vi "SaveCycleSweep.vi"(5 "Area":dbl=1.0, 6 "JunctionName":string, 7 "SideLength":dbl=1.0, 8 "UiDefinition 2":T3, 9 "InfoCluster":T1, 10 "appended array":dbl[][](array[numeric])) -> (0 "error out":errorcluster)   [LabVIEW 2020]
uses:
  UIReferences.ctl
  D:/LabviewDXFViewer/LabviewDXFViewer/bin/Release/LabviewDXFViewer.exe
  LabviewDXFViewer/bin/Release/LabviewDXFViewer.exe
  Keithley_Subs/CapacitanceInfos.ctl
  Keithley_Subs/CapacitanceRecord.ctl
  <vilib>/httpClient/POSTBuffer.vi
  <vilib>/httpClient/LabVIEWHTTPClient.lvlib
panel:
  in  "Cluster 3":T4
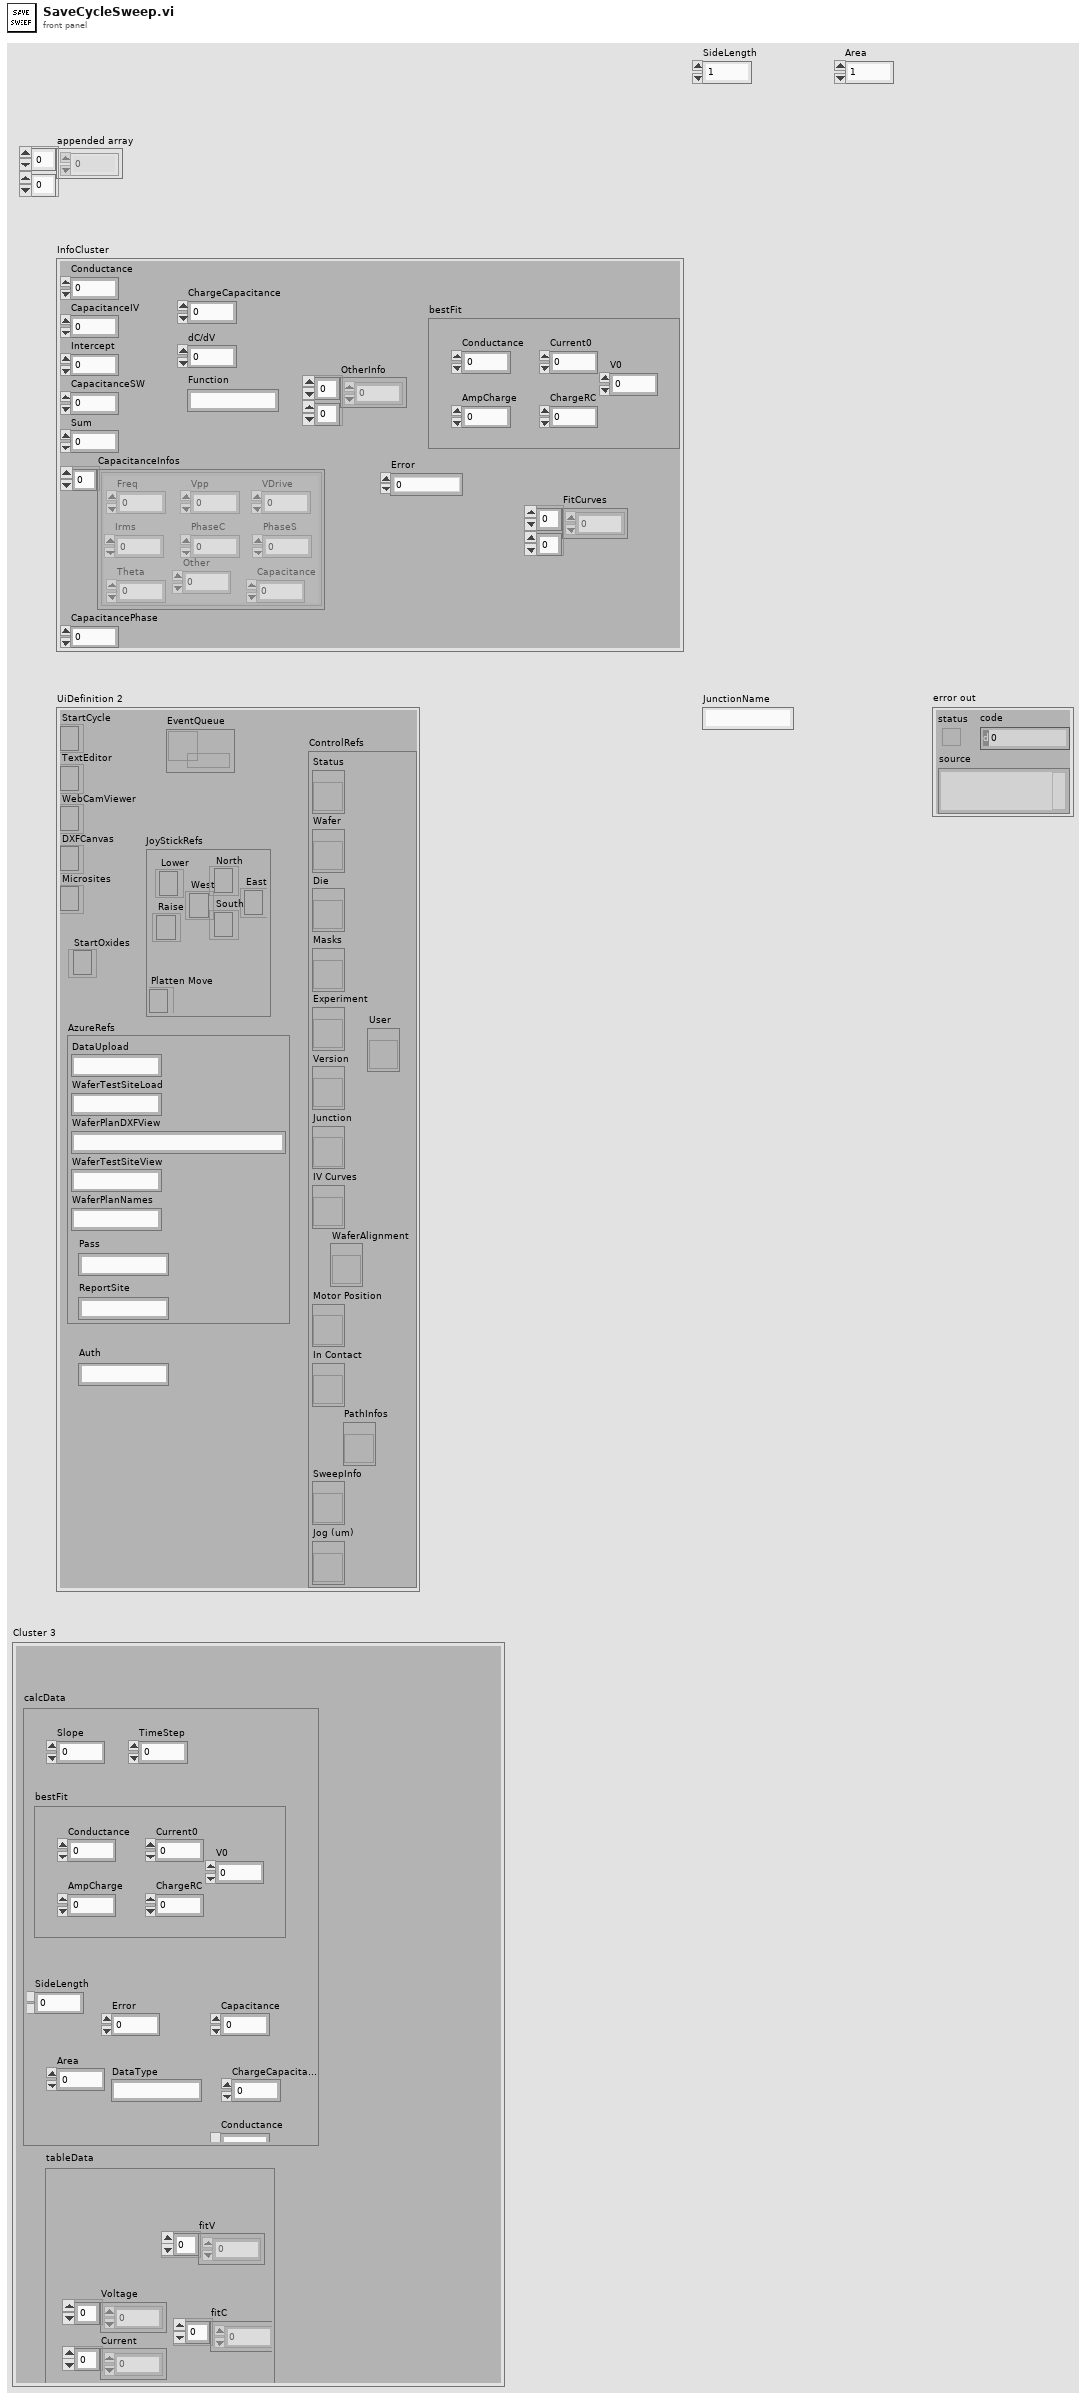
[diagram p1: front panel]
types:
  T1 = typedef "CapacitanceInfos.ctl" = cluster{"Conductance":dbl, "CapacitanceIV":dbl, "Intercept":dbl, "CapacitanceSW":dbl, "Sum":dbl, "CapacitanceInfos":T2[], "CapacitancePhase":dbl, "dC/dV":dbl, "Function":string, "OtherInfo":dbl[][], "ChargeCapacitance":dbl, "FitCurves":dbl[][], "Error":dbl, "bestFit":cluster{"Conductance":dbl, "Current0":dbl, "AmpCharge":dbl, "ChargeRC":dbl, "V0":dbl}}
  T2 = typedef "CapacitanceRecord.ctl" = cluster{"Freq":dbl, "Vpp":dbl, "PhaseS":dbl, "Irms":dbl, "PhaseC":dbl, "Theta":dbl, "VDrive":dbl, "Capacitance":dbl, "Other":dbl}
  T3 = typedef "UIReferences.ctl" = cluster{"StartCycle":refnum<k24>, "TextEditor":refnum<k24>, "WebCamViewer":refnum<k24>, "DXFCanvas":refnum<k24>, "Microsites":refnum<k24>, "JoyStickRefs":cluster{"North":refnum<k24>, "Lower":refnum<k24>, "Raise":refnum<k24>, "Platten Move":refnum<k24>, "West":refnum<k24>, "East":refnum<k24>, "South":refnum<k24>}, "AzureRefs":cluster{"DataUpload":string, "WaferTestSiteLoad":string, "WaferPlanDXFView":string, "WaferTestSiteView":string, "WaferPlanNames":string, "Pass":string, "ReportSite":string}, "ControlRefs":cluster{"Status":refnum<vi>, "Wafer":refnum<vi>, "Die":refnum<vi>, "Masks":refnum<vi>, "Experiment":refnum<vi>, "Version":refnum<vi>, "Junction":refnum<vi>, "IV Curves":refnum<vi>, "Motor Position":refnum<vi>, "In Contact":refnum<vi>, "SweepInfo":refnum<vi>, "Jog (um)":refnum<vi>, "PathInfos":refnum<vi>, "User":refnum<vi>, "WaferAlignment":refnum<vi>}, "EventQueue":refnum<queue>, "StartOxides":refnum<k24>, "Auth":string}
  T4 = cluster{"tableData":cluster{"Current":dbl[], "Voltage":dbl[], "fitV":dbl[], "fitC":dbl[]}, "calcData":cluster{"Intercept":dbl, "Slope":dbl, "Capacitance":dbl, "ChargeCapacitance":dbl, "Conductance":dbl, "Error":dbl, "Area":dbl, "SideLength":dbl, "DataType":string, "bestFit":cluster{"Conductance":dbl, "Current0":dbl, "AmpCharge":dbl, "ChargeRC":dbl, "V0":dbl}, "TimeStep":dbl}}
  T5 = cluster{"Die":string, "Wafer":string, "Path":path, "url":string, "Experiment":string, "Version":string, "user":string}
  T6 = cluster{"Conductance":dbl, "Current0":dbl, "AmpCharge":dbl, "ChargeRC":dbl, "V0":dbl}
  T7 = cluster{"Current":dbl[], "Voltage":dbl[], "fitV":dbl[], "fitC":dbl[]}
  T8 = cluster{"Intercept":dbl, "Slope":dbl, "Capacitance":dbl, "ChargeCapacitance":dbl, "Conductance":dbl, "Error":dbl, "Area":dbl, "SideLength":dbl, "DataType":string, "bestFit":cluster{"Conductance":dbl, "Current0":dbl, "AmpCharge":dbl, "ChargeRC":dbl, "V0":dbl}, "TimeStep":dbl}
  T9 = typedef "LabVIEWHTTPClient.lvlib/ClientHandle.ctl" = refnum<k1>
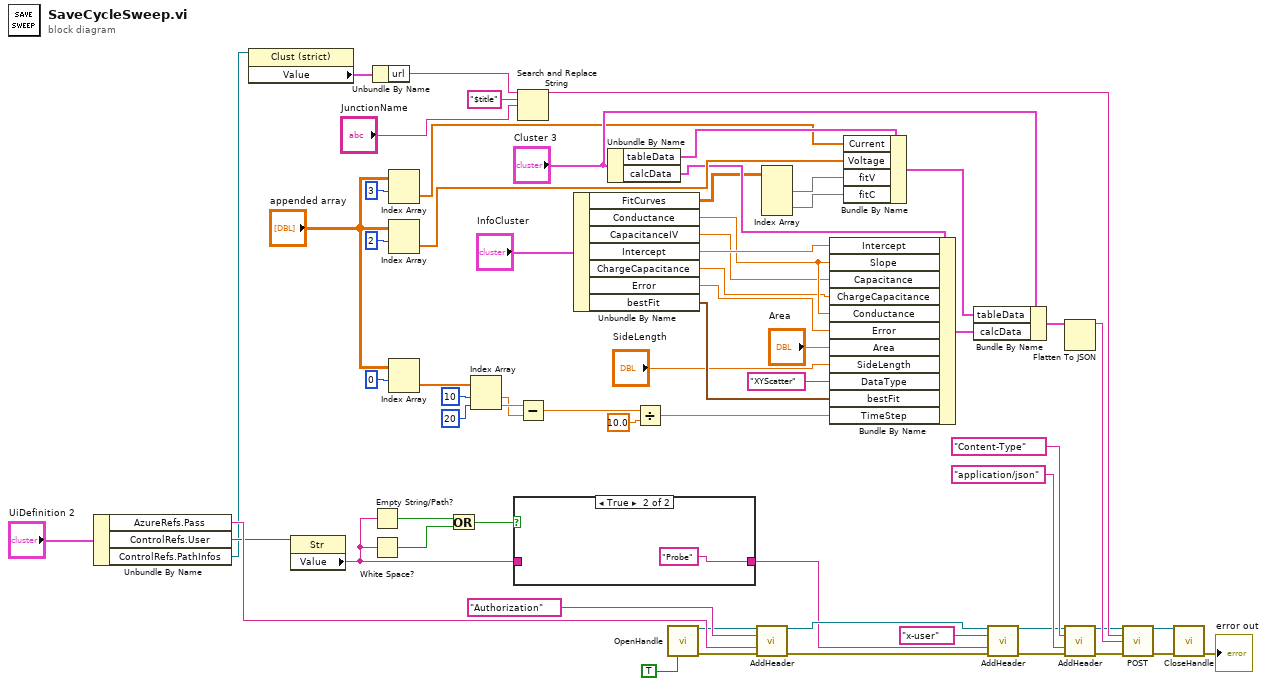
[diagram p0: block diagram]
diagram:
  n1 = Unbundle By Name("UiDefinition 2") -> ("AzureRefs.Pass"=w50:string, "ControlRefs.User"=w48:refnum<vi>, "ControlRefs.PathInfos"=w41:refnum<vi>)
  n2 = property class="Clust (strict)"(reference=w41) -> ("Value"=w40:T5)  [unwired: 1 in, 2 out]
  n3 = property class="Str"(reference=w48) -> ("Value"=w43:string)  [unwired: 1 in, 2 out]
  n4 = Empty String/Path?(string/path=w43) -> (empty?=w44:bool)
  n5 = White Space?(1:w43) -> (0:w47:bool)
  n6 = Unbundle By Name(w40) -> ("url"=w39:string)
  n7 = Index Array(array="appended array", index (row)=3) -> (element=w29:dbl[])  [unwired: 1 in]
  n8 = Index Array(array="appended array", index (row)=2) -> (element=w30:dbl[])  [unwired: 1 in]
  n9 = Index Array(array="appended array", index (row)=0) -> (element=w14:dbl[])  [unwired: 1 in]
  n10 = Or(x=w44, y=w47) -> (x .or. y?=w45:bool)
  n11 = Index Array(array=w14, index #1=10 ("index"), index #2=20 ("index")) -> (element #1=w10:dbl, element #2=w11:dbl)
  n12 = case shown="True" w45 {
    tunnel: w43 -> [w65 _]
    tunnel: [w65 "Probe"] -> w46
    frame False {
    }
    frame True {
    }
  }
  n13 = Search and Replace String(input string=w39, search string="$title" ("string"), replace string="JunctionName") -> (result string=w55:string)  [unwired: 5 in, 3 out]
  n14 = Subtract(x=w11, y=w10) -> (x-y=w9:dbl)
  n15 = Unbundle By Name("InfoCluster") -> ("FitCurves"=w1:dbl[][], "Conductance"=w17:dbl, "CapacitanceIV"=w16:dbl, "Intercept"=w21:dbl, "ChargeCapacitance"=w15:dbl, "Error"=w20:dbl, "bestFit"=w23:T6)
  n16 = Unbundle By Name("Cluster 3") -> ("tableData"=w31:T7, "calcData"=w24:T8)
  n17 = Divide(x=w9, y=10.0) -> (x/y=w7:dbl)
  n18 = call <vilib>:"OpenHandle.vi"("verify server(true)"=TRUE) -> ("client handle out"=w42:T9, "error out"=w5:errorcluster)  [unwired: 13 in]
  n19 = call <vilib>:"AddHeader.vi"("client handle"=w42, "header"="Authorization", "value"=w50, "error in (no error)"=w5) -> ("client handle out"=w52:T9, "error out"=w4:errorcluster)  [unwired: 10 in]
  n20 = Index Array(array=w1) -> (element #1=w26:dbl[], element #2=w25:dbl[])  [unwired: 4 in]
  n21 = Bundle By Name(cluster=w24, "Intercept"=w21, "Slope"=w17, "Capacitance"=w16, "ChargeCapacitance"=w15, "Conductance"=w17, "Error"=w20, "Area"="Area", "SideLength"="SideLength", "DataType"="XYScatter", "bestFit"=w23, "TimeStep"=w7) -> (w6:T8)
  n22 = Bundle By Name(cluster=w31, "Current"=w29, "Voltage"=w30, "fitV"=w26, "fitC"=w25) -> (w28:T7)
  n23 = Bundle By Name(cluster="Cluster 3", "tableData"=w28, "calcData"=w6) -> (w27:T4)
  n24 = call <vilib>:"AddHeader.vi"("client handle"=w52, "header"="x-user", "value"=w46, "error in (no error)"=w4) -> ("client handle out"=w34:T9, "error out"=w3:errorcluster)  [unwired: 10 in]
  n25 = Flatten To JSON(anything=w27) -> (JSON string=w59:string)  [unwired: 2 in, 1 out]
  n26 = call <vilib>:"AddHeader.vi"("client handle"=w34, "header"="Content-Type", "value"="application/json", "error in (no error)"=w3) -> ("client handle out"=w33:T9, "error out"=w2:errorcluster)  [unwired: 10 in]
  n27 = call-poly <vilib>:"POST.vi"("client handle"=w33, "url"=w55, "buffer"=w59, "error in (no error)"=w2) -> ("client handle out"=w58:T9, "error out"=w57:errorcluster)  [unwired: 8 in, 2 out]
  n28 = call <vilib>:"CloseHandle.vi"("client handle"=w58, "error in (no error)"=w57) -> ("error out"=→"error out":errorcluster)  [unwired: 13 in]
